vi "Write bev.vi"(8 "error in (no error)":errorcluster, 10 "Beverage.lvclass":refnum<class "Beverage.lvclass">, 11 "Vanilla in":refnum<class "Vanilla.lvclass">) -> (0 "error out":errorcluster, 3 "Vanilla out":refnum<class "Vanilla.lvclass">)   [LabVIEW 2018, in "Vanilla.lvclass"]
uses:
  Vanilla.lvclass
  Beverage Class/Beverage.lvclass
  CondimentDecorator/CondimentDecorator.lvclass
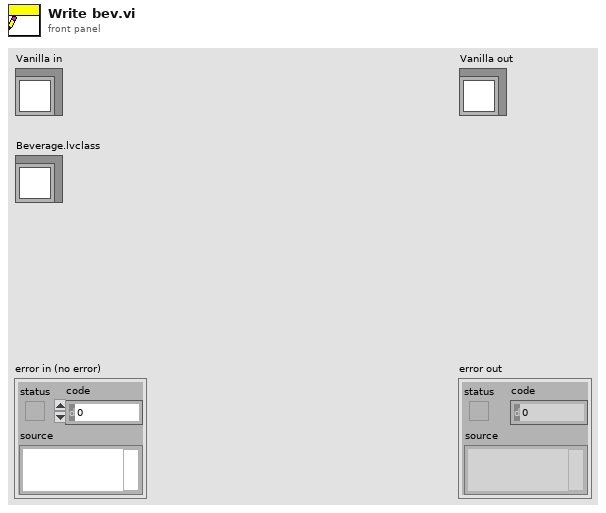
[diagram p1: front panel]
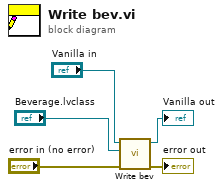
[diagram p0: block diagram]
diagram:
  n1 = call-parent "Write bev.vi"("error in (no error)"="error in (no error)", "Beverage.lvclass"="Beverage.lvclass", "CondimentDecorator in"="Vanilla in") -> ("error out"=→"error out":errorcluster, "CondimentDecorator out"=→"Vanilla out":refnum<class "Vanilla.lvclass">)  [unwired: 7 in]
